vi "decompress.vi"(8 "错误输入（无错误）":errorcluster, 11 "src":string) -> (0 "错误输出":errorcluster, 3 "dst":string)   [LabVIEW 2020, in "zstd.lvlib"]
uses:
  zstd.lvlib
  libzstd.dll
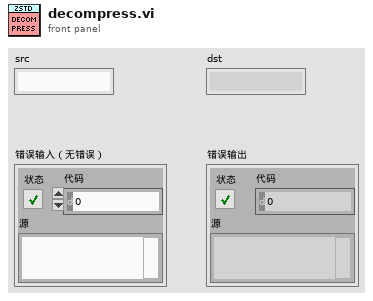
[diagram p1: front panel]
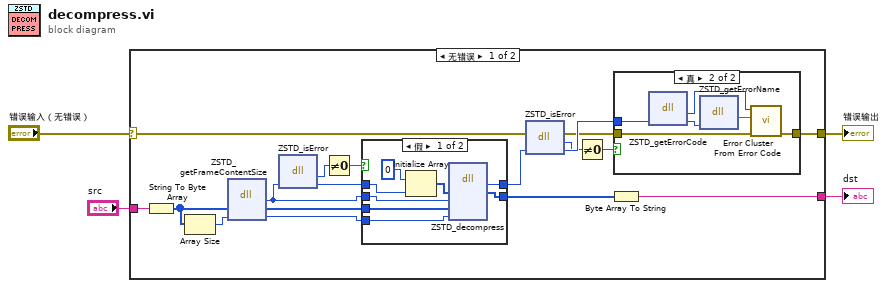
[diagram p0: block diagram]
diagram:
  n1 = case shown="无错误" "错误输入（无错误）" {
    selector: "错误输入（无错误）" -> [w10 w39]
    tunnel: "src" -> [w17 _]
    tunnel: [w16 _] -> w2
    tunnel: [w11 w39] -> w4
    frame No Error {
      n2 = String To Byte Array(string=w17) -> (unsigned byte array=w18:u8[])
      n3 = Array Size(array=w18) -> (size(s)=w19:i32)
      n4 = dll-call lib="D:/Workspace/LabVIEW/LVToolset/vi.lib/zstd/libzstd.dll" fn="ZSTD_getFrameContentSize"("src"=w18, "srcSize"=w19) -> ("return"=w8:u32, "src"=w22:u8[], "srcSize"=w21:u32)  [unwired: 3 in, 2 out]
      n5 = dll-call lib="D:/Workspace/LabVIEW/LVToolset/vi.lib/zstd/libzstd.dll" fn="ZSTD_isError"("result"=w8) -> ("return"=w6:u8, "result"=w7:u32)  [unwired: 3 in, 2 out]
      n6 = Not Equal To 0?(x=w6) -> (x != 0?=w5:bool)
      n7 = case shown="假" w5 {
        tunnel: w22 -> [w28 _]
        tunnel: w21 -> [w27 _]
        tunnel: [w26 _] -> w20
        tunnel: [w25 w31] -> w12
        tunnel: w8 -> [w24 _]
        tunnel: w7 -> [w23 w31]
        frame False {
          n8 = Initialize Array(u8 0 ("无符号8位整型"), w23) -> (w29:u8[])
          n9 = dll-call lib="D:/Workspace/LabVIEW/LVToolset/vi.lib/zstd/libzstd.dll" fn="ZSTD_decompress"("dst"=w29, "dstCapacity"=w24, "src"=w28, "compressedSize"=w27) -> ("return"=w25:u32, "dst"=w26:u8[])  [unwired: 6 in, 2 out]
        }
        frame True {
        }
      }
      n10 = dll-call lib="D:/Workspace/LabVIEW/LVToolset/vi.lib/zstd/libzstd.dll" fn="ZSTD_isError"(error in=w10, "result"=w12) -> (error out=w9:errorcluster, "return"=w14:u8, "result"=w15:u32)  [unwired: 2 in, 1 out]
      n11 = Not Equal To 0?(x=w14) -> (x != 0?=w13:bool)
      n12 = Byte Array To String(unsigned byte array=w20) -> (string=w16:string)
      n13 = case shown="真" w13 {
        tunnel: w15 -> [_ w38]
        tunnel: [w32 w34] -> w11
        tunnel: w9 -> [w32 w33]
        frame False {
        }
        frame True {
          n14 = dll-call lib="D:/Workspace/LabVIEW/LVToolset/vi.lib/zstd/libzstd.dll" fn="ZSTD_getErrorCode"("functionResult"=w38) -> ("return"=w35:i32, "functionResult"=w37:u32)  [unwired: 3 in, 2 out]
          n15 = dll-call lib="D:/Workspace/LabVIEW/LVToolset/vi.lib/zstd/libzstd.dll" fn="ZSTD_getErrorName"("code"=w37) -> ("return"=w36:string)  [unwired: 4 in, 2 out]
          n16 = call <vilib>:"Error Cluster From Error Code.vi"("error in (no error)"=w33, "error message (\"\")"=w36, "error code (0)"=w35) -> ("error out"=w34:errorcluster)  [unwired: 6 in]
        }
      }
    }
    frame Error {
    }
  }
  "错误输出" <- w4
  "dst" <- w2
